vi "Register gRPC Methods.vi"(8 "error in (no error)":errorcluster, 11 "Template Server in":refnum<class "server12.lvclass">) -> (0 "error out":errorcluster, 3 "Template Server out":refnum<class "server12.lvclass">)   [LabVIEW 2020, in "server12.lvlib" / "server12.lvclass"]
uses:
  server12.lvclass
  server12.lvclass/server12.ctl
  typeDefs/Server Internal UEs.ctl
  typeDefs/Server gRPC UEs.ctl
  gRPC lvSupport/Server API/typeDefs/grpcId.ctl
  gRPC lvSupport/gprc-lvsupport.lvlib
  gRPC lvSupport/Server API/typeDefs/gRPCId Cluster.ctl
  typeDefs/Server Internal Message.ctl
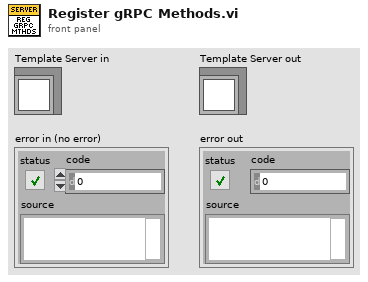
[diagram p1: front panel]
types:
  T1 = typedef "server12.lvlib/server12.lvclass/Server gRPC UEs.ctl" = cluster{"getCANDatafromrgrpcServer_clientRequester_getIDFormServer gRPC UE":refnum<user-event>}
  T2 = typedef "server12.lvlib/server12.lvclass/Server Internal UEs.ctl" = cluster{"getCANDatafromrgrpcServer_clientRequester_getIDFormServer Internal UE":refnum<user-event>}
  T3 = typedef "server12.lvlib/gprc-lvsupport.lvlib/grpcId.ctl" = u64
  T4 = typedef "server12.lvlib/server12.lvclass/Server Internal Message UE.ctl" = refnum<user-event>
  T5 = typedef "server12.lvlib/gprc-lvsupport.lvlib/gRPCId Cluster UE.ctl" = refnum<user-event>
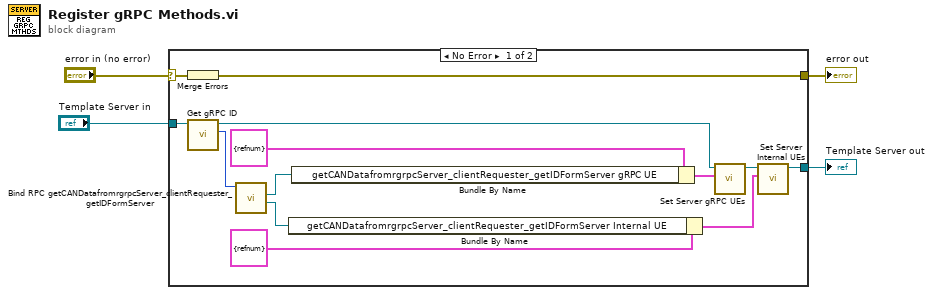
[diagram p0: block diagram]
diagram:
  n1 = case shown="No Error" "error in (no error)" {
    selector: "error in (no error)" -> [w8 w18]
    tunnel: "Template Server in" -> [w16 w19]
    tunnel: [w15 w18] -> w3
    tunnel: [w14 w19] -> w2
    frame No Error {
      n2 = Merge Errors(w8) -> (w15:errorcluster)
      n3 = call "Get gRPC ID.vi"("OOP Server in"=w16) -> ("gRPC ID"=w7:T3, "OOP Server out"=w17:refnum<class "server12.lvclass">)  [unwired: 9 in]
      n4 = call "Bind RPC getCANDatafromrgrpcServer_clientRequester_getIDFormServer.vi"("gRPCid server in"=w7) -> ("getCANDatafromrgrpcServer_clientRequester_getIDFormServer Internal UE"=w6:T4, "getCANDatafromrgrpcServer_clientRequester_getIDFormServer gRPC UE"=w5:T5)  [unwired: 7 in, 2 out]
      n5 = Bundle By Name ("Bundle Internal UEs")(cluster=T2 {"getCANDatafromrgrpcServer_clientRequester_getIDFormServer Internal UE"=refnum} ("Server Internal UEs"), "getCANDatafromrgrpcServer_clientRequester_getIDFormServer Internal UE"=w6) -> (w13:T2)
      n6 = Bundle By Name ("Bundle gRPC UEs")(cluster=T1 {"getCANDatafromrgrpcServer_clientRequester_getIDFormServer gRPC UE"=refnum} ("gRPC Server Method Events"), "getCANDatafromrgrpcServer_clientRequester_getIDFormServer gRPC UE"=w5) -> (w10:T1)
      n7 = call "Set Server gRPC UEs.vi"("Server gRPC UEs"=w10, "OOP Server in"=w17) -> ("OOP Server out"=w11:refnum<class "server12.lvclass">)  [unwired: 9 in]
      n8 = call "Set Server Internal UEs.vi"("Server Internal UEs"=w13, "OOP Server in"=w11) -> ("OOP Server out"=w14:refnum<class "server12.lvclass">)  [unwired: 9 in]
    }
    frame Error {
    }
  }
  "error out" <- w3
  "Template Server out" <- w2
